vi "UDP Buffered Tx Process.vi"(10 "Parameters":variant, 11 "Process":refnum<class "Process.lvclass">) -> ()   [LabVIEW 2016, in "UDP-Custom-Device Engine.lvlib"]
uses:
  UDP-Custom-Device Engine.lvlib
  <vilib>/NI/NIVS Inline Async API/_VS Inline Async API/Process/Process.lvclass
  <vilib>/NI/NIVS Inline Async API/_VS Inline Async API/Process/Process.lvclass/Process.ctl
  <vilib>/NI/NIVS Inline Async API/_Data Access Engine/Access Type Classes/Read/Read.lvclass/Read.ctl
  <vilib>/NI/NIVS Inline Async API/_Data Access Engine/Access Type Classes/Write/Write.lvclass/Write.ctl
  <vilib>/NI/NIVS Inline Async API/_VS Inline Async API/Process/Data Member Access/Read Data Access.vi
  <vilib>/NI/NIVS Inline Async API/_VS Inline Async API/Error Handling Process/SubVIs/Error.ConvertArray.vi
  Buffered Transmit/Run Bfr Tx - Handle Transmit Size.vi
  Transmit/Run Tx - Handle Port Tx Check.vi
  <vilib>/NI/NIVS Inline Async API/_Data Access Engine/Data Access Engine/Methods/Data.Processes.Execute.vi
  <vilib>/NI/NIVS Inline Async API/_Data Access Engine/Data Access Engine/Methods/Write.Data.vi
  <vilib>/NI Veristand/VeriStand Data/Pointer Operations/Pointer.In-Place Read.vi
  <vilib>/NI Veristand/VeriStand Data/Pointer Operations/Pointer.In-Place Read (1D U8).vi
  Buffered Transmit/Run Bfr Tx - FIFO Entry Size.vi
  Buffered Transmit/Run Bfr Tx - FIFO Payload.vi
  Buffered Transmit/Run Bfr Tx - FIFO Count Packets.vi
  <vilib>/NI/NIVS Inline Async API/_Data Access Engine/Data Access Engine/Methods/Read.Data.vi
  <vilib>/NI Veristand/VeriStand Data/Type Conversion/Type Conversion.From Double.vi
  <vilib>/NI Veristand/VeriStand Data/Type Conversion/Type Conversion.From Double (I32).vi
  <vilib>/NI/NIVS Inline Async API/_Data Access Engine/Access Type Classes/Write/Write.ProcessData.vi
  <vilib>/NI Veristand/VeriStand Data/Pointer Operations/Pointer.Read.vi
  <vilib>/NI Veristand/VeriStand Data/Pointer Operations/Pointer.Read (I32).vi
  <vilib>/NI/NIVS Inline Async API/_Data Access Engine/Access Type Classes/Read/Read.ProcessData.vi
  <vilib>/NI Veristand/VeriStand Data/Pointer Operations/Pointer.In-Place Read (I32).vi
  Buffered Transmit/Run Bfr Tx - FIFO Port.vi
  Transmit/Run Tx - Handle Transmit Option.vi
  <vilib>/NI/NIVS Inline Async API/_Data Access Engine/Data Access Engine/Data Access Engine.lvclass
  <vilib>/NI Veristand/VeriStand Data/VeriStand Data.lvlib
panel:
  out "Data Buffer":u64 format="%016x"
  out "Tx Packet":string
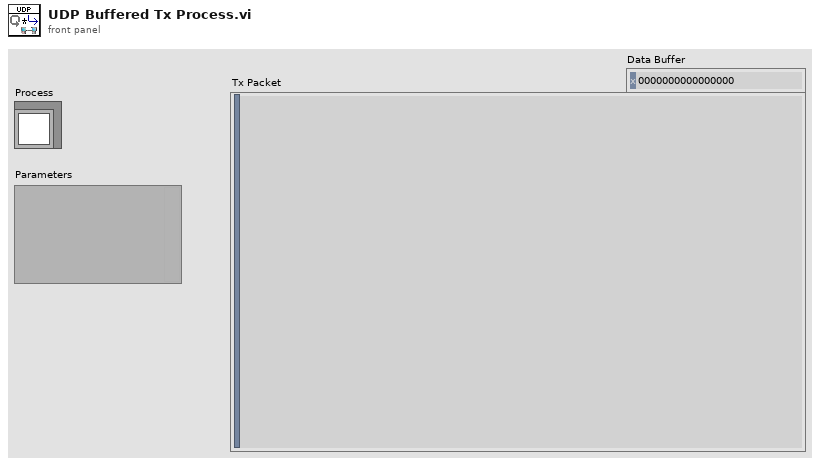
[diagram p1: front panel]
types:
  T1 = typedef "UDP-Custom-Device Engine.lvlib/Engine - Buffered Tx Loop Data.ctl" = cluster{"General Resources":T2, "Header Details":T4, "Buffer Resources":T5, "Runtime Resources":T7, "Echo Resources":T9, "Buffer Option Support":T11, "Channel Resources":T14, "Debug Resources":T17}
  T2 = typedef "UDP-Custom-Device Engine.lvlib/Engine - General Resources.ctl" = cluster{"Packet Name":string, "Packet ID":i32, "Local IP Address":string, "Local Port":i32, "Multicast":bool, "Multicast IP Address":u32, "Header Info":bool[], "Byte Order":enum16{"big-endian, network order", "native, host order", "little-endian"}, "Channel Data Types":T3[], "Duplex Packets":refnum<data-value>}
  T3 = typedef "VeriStand Data.lvlib/Typedefs.Data Types.ctl" = enum16{"Boolean", "Single", "Double", "I8", "I16", "I32", "I64", "U8", "U16", "U32", "U64"}
  T4 = typedef "UDP-Custom-Device Shared.lvlib/Shared - Header Details.ctl" = cluster{"Packet Size":u16, "Protocol Revision":u8, "System Definition Version":u64, "Source Node Name":string, "Packet ID":u32, "Number of Channels":u32, "Static Header Size":u16, "Total Header Size":u16}
  T5 = typedef "UDP-Custom-Device Engine.lvlib/Engine - Buffer Resources.ctl" = cluster{"Data Buffer":u64, "Pointer Encoding":T6, "Buffer Size":i32, "Raw Buffer Data":u8[], "Is Buffered":bool, "External Buffer":bool, "Prepend Header":bool, "Valid Buffer":bool}
  T6 = typedef "UDP-Custom-Device Shared.lvlib/Shared - Pointer Encoding.ctl" = enum16{"Direct Encoding", "Conversion Encoding"}
  T7 = typedef "UDP-Custom-Device Engine.lvlib/Engine - Tx Runtime Resources.ctl" = cluster{"Connection ID":refnum<k16>, "Transmit Option":T8, "Destination IP Address":u32, "Destination Port":u16, "Multicast IP Address":u32, "TTL":u16, "Multicast":bool, "Port as Channel":bool, "Loop Period":u32, "Target Processor":i32, "Priority":i32}
  T8 = typedef "UDP-Custom-Device Shared.lvlib/Shared - Transmit Flag Options.ctl" = enum16{"Always", "One-Shot", "Toggle"}
  T9 = typedef "UDP-Custom-Device Engine.lvlib/Engine - Tx Echo Resources.ctl" = cluster{"Transmit Echo Option":T10, "Packet Count":dbl, "Counter Increment":dbl, "Transmit Values":dbl[]}
  T10 = typedef "UDP-Custom-Device Shared.lvlib/Shared - Transmit Echo Options.ctl" = enum16{"PCL Reset", "Counter", "Mirror"}
  T11 = typedef "UDP-Custom-Device Engine.lvlib/Engine - Buffered Tx Buffer Option Support.ctl" = cluster{"Buffer Option":T12, "Sim Option":T13}
  T12 = typedef "UDP-Custom-Device Shared.lvlib/Shared - Transmit Buffer Options.ctl" = enum16{"Static Buffer", "FIFO Buffer", "FIFO Buffer + Port"}
  T13 = typedef "UDP-Custom-Device Shared.lvlib/Shared - Transmit Sim Options.ctl" = enum16{"No Simulation", "Counter", "Full Buffer", "FIFO Test", "FIFO + Port Test"}
  T14 = typedef "UDP-Custom-Device Engine.lvlib/Engine - Buffered Tx Channel Refs.ctl" = cluster{"Transmit Flag":T15, "Transmit Echo":T16, "Transmit Bytes":T15, "Port Channel":T15, "Buffer (External)":T15, "Buffer (Local)":T16, "Timestamp":T15}
  T15 = typedef "Data Access Engine.lvlib/Data Access Engine.lvclass/Read.DVR.ctl" = refnum<data-value>
  T16 = typedef "Data Access Engine.lvlib/Data Access Engine.lvclass/Write.DVR.ctl" = refnum<data-value>
  T17 = typedef "UDP-Custom-Device Engine.lvlib/Engine - Debug Resources.ctl" = cluster{"Debug Mode":bool, "Debug Log File":refnum<file>, "Packet Name":string}
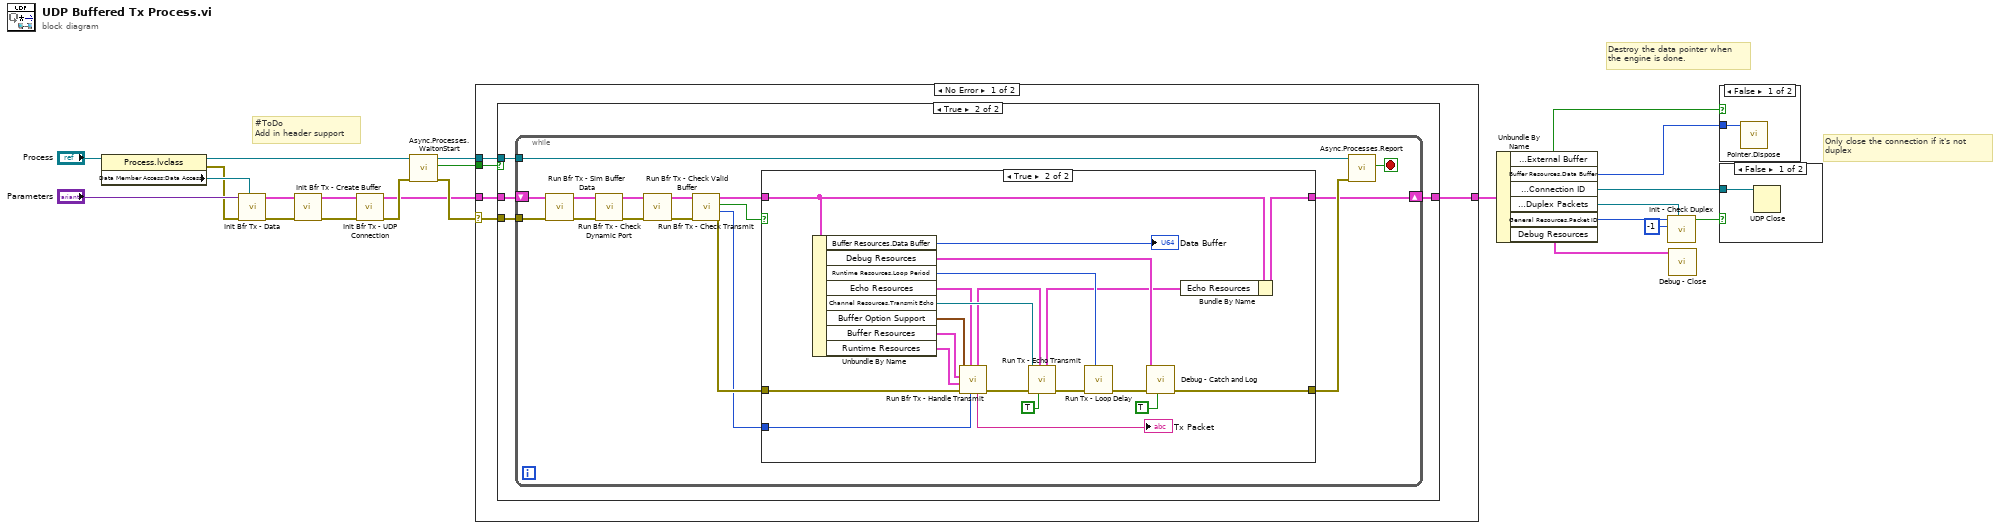
[diagram p0: block diagram]
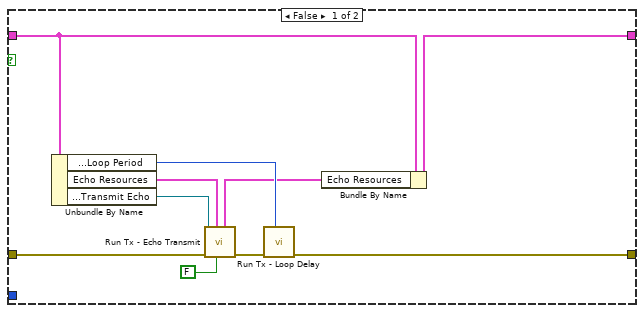
[diagram p3: hidden frame]
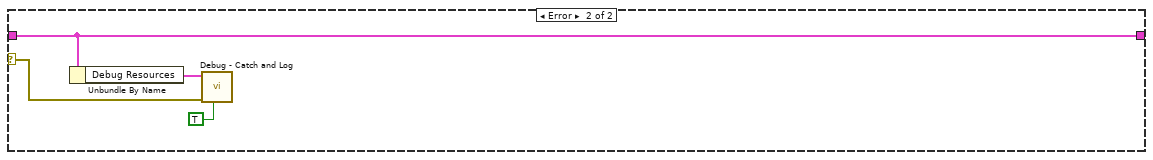
[diagram p4: hidden frame]
diagram:
  # "Only close the connection if it's not\nduplex"
  # "Destroy the data pointer when\nthe engine is done."
  # "#ToDo\nAdd in header support"
  n1 = property class="Process.lvclass"(reference="Process") -> (reference out=w23:refnum<class "Process.lvclass">, error out=w15:errorcluster, "Data Member Access:Data Access"=w16:refnum<class "Data Access Engine.lvclass">)  [unwired: 1 in]
  n2 = call "Init Bfr Tx - Data.vi"("Data Access"=w16, "error in (no error)"=w15, "Parameters"="Parameters") -> ("error out"=w13:errorcluster, "Tx Loop Data"=w14:T1)  [unwired: 7 in]
  n3 = call "Init Bfr Tx - Create Buffer.vi"("error in (no error)"=w13, "Tx Loop Data in"=w14) -> ("error out"=w11:errorcluster, "Tx Loop Data out"=w12:T1)  [unwired: 8 in]
  n4 = call "Init Bfr Tx - UDP Connection.vi"("error in (no error)"=w11, "Tx Loop Data in"=w12) -> ("error out"=w10:errorcluster, "Tx Loop Data out"=w8:T1)  [unwired: 8 in]
  n5 = call <vilib>:"Async.Processes.WaitonStart.vi"("error in (no error)"=w10, "Process"=w23) -> ("error out"=w21:errorcluster, "Execute"=w19:bool, "Process out"=w20:refnum<class "Process.lvclass">)  [unwired: 7 in]
  n6 = case shown="No Error" w21 {
    selector: w21 -> [w26 w83]
    tunnel: w19 -> [w28 _]
    tunnel: w20 -> [w27 _]
    tunnel: w8 -> [w25 w81]
    tunnel: [w24 w81] -> w18
    frame No Error {
      n7 = case shown="True" w28 {
        tunnel: w26 -> [_ w32]
        tunnel: w27 -> [_ w33]
        tunnel: w25 -> [w29 w31]
        tunnel: [w29 w30] -> w24
        frame False {
        }
        frame True {
          n8 = while {
            tunnel: w32 -> [w45]
            tunnel: w33 -> [w49]
            shift-right: [w44] -> w30
            shift-left: w31 -> [w46]
            stop <- w48 stop-if-true
            n9 = call "Run Bfr Tx - Sim Buffer Data.vi"("error in (no error)"=w45, "Tx Loop Data in"=w46) -> ("error out"=w35:errorcluster, "Tx Loop Data out"=w37:T1)  [unwired: 8 in]
            n10 = call "Run Bfr Tx - Check Dynamic Port.vi"("error in (no error)"=w35, "Tx Loop Data in"=w37) -> ("error out"=w34:errorcluster, "Tx Loop Data out"=w36:T1)  [unwired: 8 in]
            n11 = call "Run Bfr Tx - Check Valid Buffer.vi"("error in (no error)"=w34, "Tx Loop Data in"=w36) -> ("error out"=w38:errorcluster, "Tx Loop Data out"=w39:T1)  [unwired: 8 in]
            n12 = call "Run Bfr Tx - Check Transmit.vi"("error in (no error)"=w38, "Tx Loop Data in"=w39) -> ("error out"=w43:errorcluster, "Bytes to Transmit"=w40:i32, "Transmit?"=w42:bool, "Tx Loop Data out"=w41:T1)  [unwired: 6 in]
            n13 = case shown="True" w42 {
              tunnel: [w56 w72] -> w47
              tunnel: [w52 w75] -> w44
              tunnel: w43 -> [w58 w69]
              tunnel: w41 -> [w53 w76]
              tunnel: w40 -> [_ w65]
              frame False {
                n14 = Unbundle By Name(w53) -> ("Runtime Resources.Loop Period"=w55:u32, "Echo Resources"=w51:T9, "Channel Resources.Transmit Echo"=w59:T16)
                n15 = call "Run Tx - Echo Transmit.vi"("Transmitted?"=FALSE, "Echo Resources in"=w51, "error in (no error)"=w58, "Ref"=w59) -> ("error out"=w57:errorcluster, "Echo Resources out"=w50:T9)  [unwired: 6 in]
                n16 = call "Run Tx - Loop Delay.vi"("Delay (ms)"=w55, "error in (no error)"=w57) -> ("error out"=w56:errorcluster)  [unwired: 9 in]
                n17 = Bundle By Name(cluster=w53, "Echo Resources"=w50) -> (w52:T1)
              }
              frame True {
                n18 = Unbundle By Name(w76) -> ("Buffer Resources.Data Buffer"=→"Data Buffer":u64, "Debug Resources"=w71:T17, "Runtime Resources.Loop Period"=w78:u32, "Echo Resources"=w61:T9, "Channel Resources.Transmit Echo"=w80:T16, "Buffer Option Support"=w62:T11, "Buffer Resources"=w63:T5, "Runtime Resources"=w64:T7)
                n19 = call "Run Bfr Tx - Handle Transmit.vi"("Bytes to Transmit"=w65, "Echo Resources in"=w61, "error in (no error)"=w69, "Runtime Resources"=w64, "Buffer Resources"=w63, "Buffer Option Support in"=w62) -> ("error out"=w68:errorcluster, "Tx Packet"=→"Tx Packet":string, "Echo Resources out"=w60:T9)  [unwired: 3 in]
                n20 = call "Run Tx - Echo Transmit.vi"("Transmitted?"=TRUE, "Echo Resources in"=w60, "error in (no error)"=w68, "Ref"=w80) -> ("error out"=w79:errorcluster, "Echo Resources out"=w70:T9)  [unwired: 6 in]
                n21 = call "Run Tx - Loop Delay.vi"("Delay (ms)"=w78, "error in (no error)"=w79) -> ("error out"=w73:errorcluster)  [unwired: 9 in]
                n22 = call "Debug - Catch and Log.vi"("Clear Error?"=TRUE, "error in (no error)"=w73, "Debug Resources"=w71) -> ("error out"=w72:errorcluster)  [unwired: 8 in]
                n23 = Bundle By Name(cluster=w76, "Echo Resources"=w70) -> (w75:T1)
              }
            }
            n24 = call <vilib>:"Async.Processes.Report.vi"("Error"=w47, "Process in"=w49) -> ("Stop"=w48:bool)  [unwired: 8 in, 1 out]
          }
        }
      }
    }
    frame Error {
      n25 = Unbundle By Name(w81) -> ("Debug Resources"=w82:T17)
      n26 = call "Debug - Catch and Log.vi"("Clear Error?"=TRUE, "error in (no error)"=w83, "Debug Resources"=w82) -> ()  [unwired: 8 in, 1 out]
    }
  }
  n27 = Unbundle By Name(w18) -> ("Buffer Resources.External Buffer"=w7:bool, "Buffer Resources.Data Buffer"=w9:u64, "Runtime Resources.Connection ID"=w2:refnum<k16>, "General Resources.Duplex Packets"=w5:refnum<data-value>, "General Resources.Packet ID"=w4:i32, "Debug Resources"=w1:T17)
  n28 = call "Init - Check Duplex.vi"("Duplex Packets"=w5, "Receive Packet ID"=-1, "Transmit Packet ID"=w4) -> ("Is Duplex?"=w3:bool)  [unwired: 6 in, 2 out]
  n29 = call "Debug - Close.vi"("Debug Resources"=w1) -> ()  [unwired: 10 in, 1 out]
  n30 = case shown="False" w7 {
    tunnel: w9 -> [w85 _]
    frame False {
      n31 = call <vilib>:"Pointer.Dispose.vi"("pointer"=w85) -> ()  [unwired: 9 in, 2 out]
    }
    frame True {
    }
  }
  n32 = case shown="False" w3 {
    tunnel: w2 -> [w86 _]
    frame False {
      n33 = UDP Close(connection ID=w86) -> ()  [unwired: 1 in, 2 out]
    }
    frame True {
    }
  }
